vi "Decode Data Stream.vi"(8 "error in (no error)":errorcluster, 10 "string":string, 11 "CR5 Data in":refnum<class "CR5 Data.lvclass">) -> (0 "error out":errorcluster, 3 "CR5 Data out":refnum<class "CR5 Data.lvclass">)   [LabVIEW 2015, in "CR5 Data.lvclass"]
uses:
  CR5 Data.lvclass
  <vilib>/Utility/miscctls.llb/LVDateTimeRec.ctl
  CR5 Data.lvclass/CR5 Data.ctl
  Accessors/Write Balance.vi
  Accessors/Write Tamb.vi
  Accessors/Write Tmirror.vi
  Accessors/Write flag.vi
  Accessors/Write PWM.vi
  Accessors/Write mirror flag.vi
  Accessors/Write Tboard.vi
  Reusable/Data/Write measTime.vi
panel:
  out "array":string[](array[string])
  out "trimmed string":string
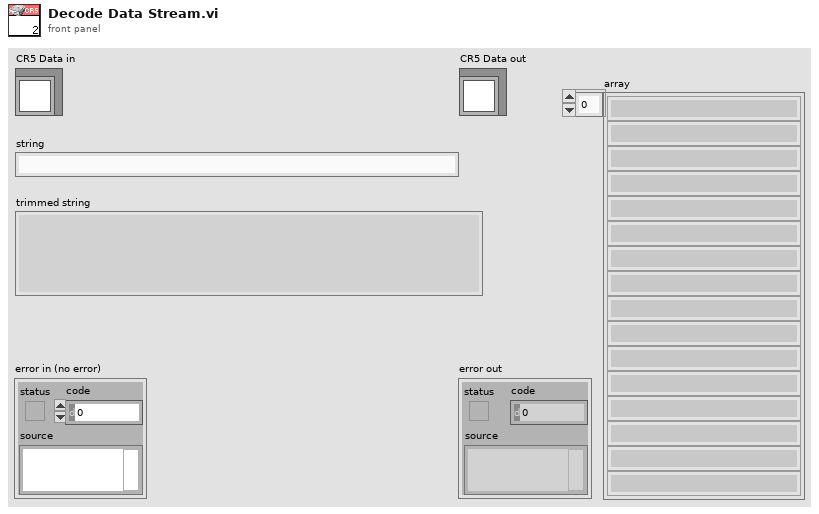
[diagram p1: front panel]
types:
  T1 = typedef "LVDateTimeRec.ctl" = cluster{"fractional second":dbl, "second":i32, "minute":i32, "hour":i32, "day of month":i32, "month":i32, "year":i32, "day of week":i32, "day of year":i32, "DST":i32}
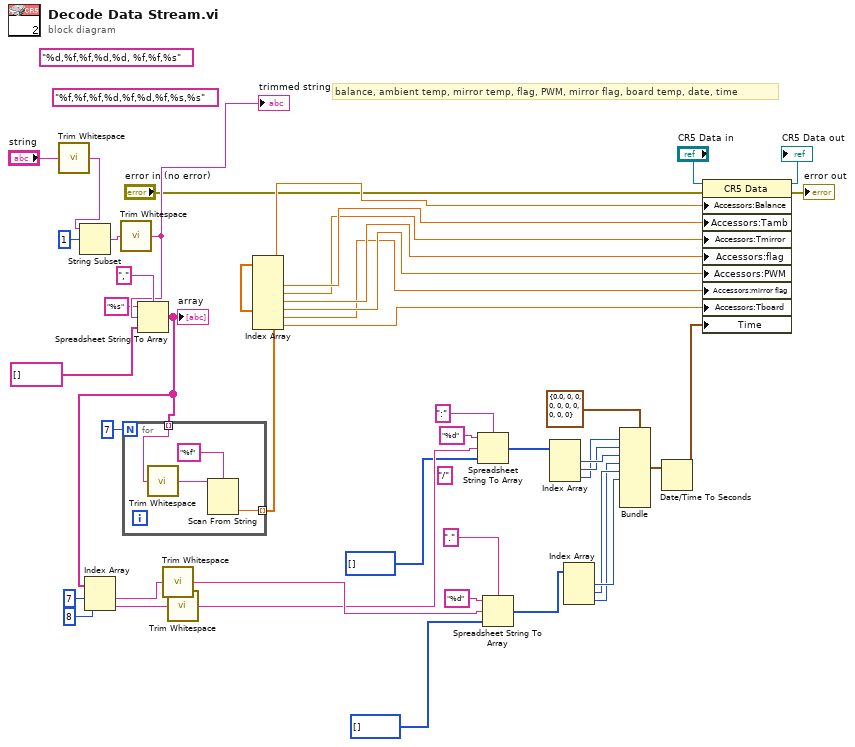
[diagram p0: block diagram]
diagram:
  (unwired) "/" ("delimiter (Tab)")
  (unwired) "%d,%f,%f,%d,%d, %f,%f,%s" ("format string")
  (unwired) "%f,%f,%f,%d,%f,%d,%f,%s,%s" ("format string")
  # "balance, ambient temp, mirror temp, flag, PWM, mirror flag, board temp, date, time"
  n1 = call <vilib>:"Trim Whitespace.vi"("string"="string") -> ("trimmed string"=w39:string)  [unwired: 1 in]
  n2 = String Subset(string=w39, offset (0)=1) -> (substring=w38:string)  [unwired: 1 in]
  n3 = call <vilib>:"Trim Whitespace.vi"("string"=w38) -> ("trimmed string"=w35:string)  [unwired: 1 in]
  "trimmed string" <- w35
  n4 = Spreadsheet String To Array(delimiter (Tab)=",", format string="%s", spreadsheet string=w35, array type (2D Dbl)=string[] []) -> (array=w32:string[])
  "array" <- w32
  n5 = Index Array(array=w32, index #1=7 ("index"), index #2=8 ("index")) -> (element #1=w29:string, element #2=w28:string)
  n6 = for {
    N: 7 -> [_]
    tunnel: w32 -> [w49] mode=indexing
    tunnel: [w46] -> w27 mode=indexing
    n7 = call <vilib>:"Trim Whitespace.vi"("string"=w49) -> ("trimmed string"=w48:string)  [unwired: 1 in]
    n8 = Scan From String(format string="%f", input string=w48) -> (output 1=w46:dbl)  [unwired: 3 in, 3 out]
  }
  n9 = call <vilib>:"Trim Whitespace.vi"("string"=w29) -> ("trimmed string"=w18:string)  [unwired: 1 in]
  n10 = call <vilib>:"Trim Whitespace.vi"("string"=w28) -> ("trimmed string"=w17:string)  [unwired: 1 in]
  n11 = Index Array(array=w27) -> (element #1=w26:dbl, element #2=w25:dbl, element #3=w24:dbl, element #4=w23:dbl, element #5=w22:dbl, element #6=w21:dbl, element #7=w20:dbl)  [unwired: 7 in]
  n12 = Spreadsheet String To Array(delimiter (Tab)=":", format string="%d", spreadsheet string=w17, array type (2D Dbl)=i32[] []) -> (array=w8:i32[])
  n13 = Spreadsheet String To Array(delimiter (Tab)=".", format string="%d", spreadsheet string=w18, array type (2D Dbl)=i32[] []) -> (array=w4:i32[])
  n14 = Index Array(array=w8) -> (element #1=w14:i32, element #2=w13:i32, element #3=w12:i32)  [unwired: 3 in]
  n15 = Index Array(array=w4) -> (element #1=w3:i32, element #2=w2:i32, element #3=w1:i32)  [unwired: 3 in]
  n16 = Bundle(cluster=T1 {"fractional second"=0.0, "second"=0, "minute"=0, "hour"=0, "day of month"=0, "month"=0, "year"=0, "day of week"=0, "day of year"=0, "DST"=0} ("date time rec"), "second"=w12, "minute"=w13, "hour"=w14, "day of month"=w1, "month"=w2, "year"=w3) -> (w15:T1)  [unwired: 4 in]
  n17 = Date/Time To Seconds(2:w15) -> (0:w41:timestamp)  [unwired: 1 in]
  n18 = property class="CR5 Data"(reference="CR5 Data in", error in="error in (no error)", "Accessors:Balance"=w26, "Accessors:Tamb"=w25, "Accessors:Tmirror"=w24, "Accessors:flag"=w23, "Accessors:PWM"=w22, "Accessors:mirror flag"=w21, "Accessors:Tboard"=w20, "Time"=w41) -> (reference out=→"CR5 Data out":refnum<class "CR5 Data.lvclass">, error out=→"error out":errorcluster)
